vi "Path to L5K to import.vi"(8 "error in (no error)":errorcluster) -> (2 "Cancelled?":bool, 3 "Path to L5K file to import out":path)   [LabVIEW 2010, in "Ethernet IP Custom Device Custom Device.lvlib"]
doc: "Use this template to create a dialog box with event handling."
uses:
  Ethernet IP Custom Device Custom Device.lvlib
  <vilib>/NI VeriStand/Custom Device API/Custom Device Item Ref.ctl
  Ethernet IP Global Strings.vi
  <vilib>/NI Veristand/Custom Device API/Custom Device API.lvlib
panel:
  out "error out":errorcluster
  in  "Node Ptr":T1 format="%.0x"
  in  "Path to L5K file to import":path
  in  "Cancel":bool
  in  "OK":bool
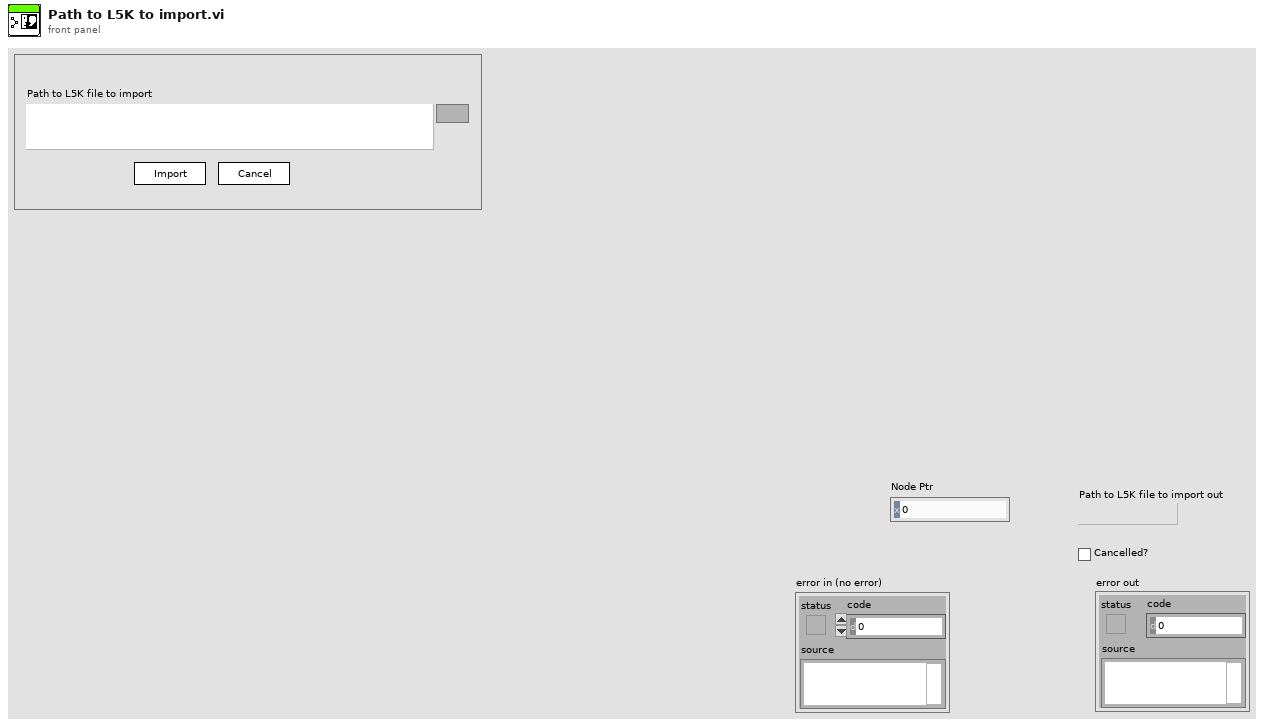
[diagram p1: front panel]
types:
  T1 = typedef "Custom Device API.lvlib/Custom Device Item Ref.ctl" = u64
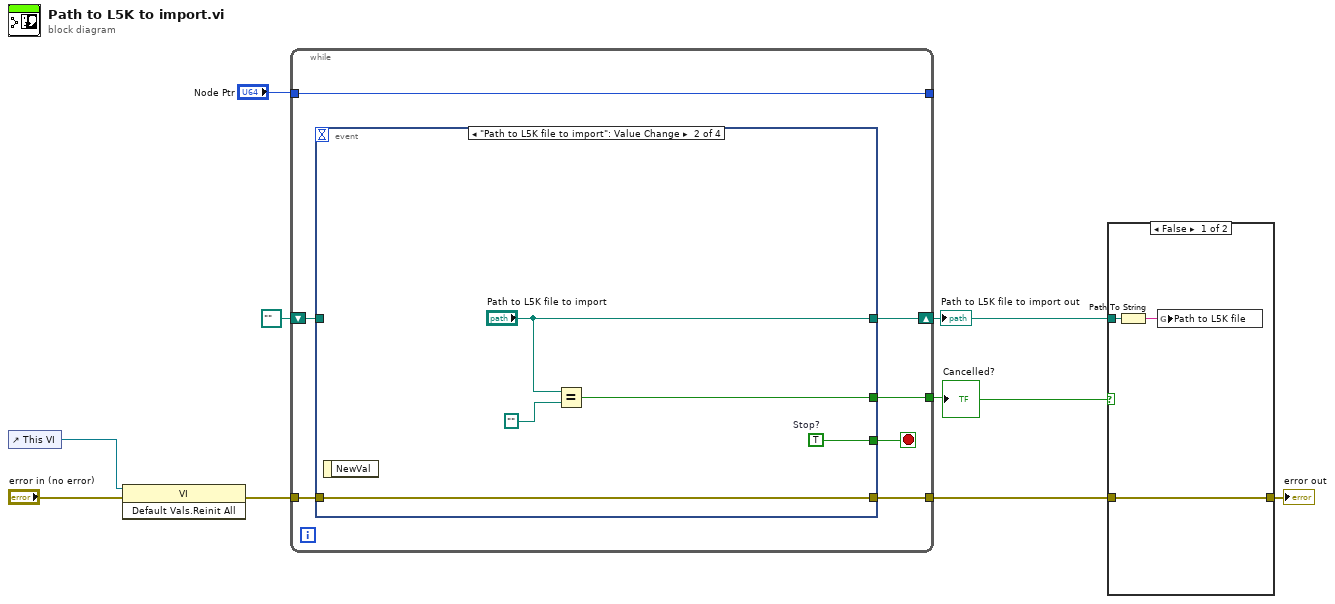
[diagram p0: block diagram]
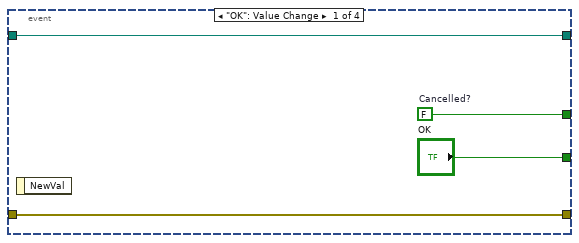
[diagram p3: hidden frame]
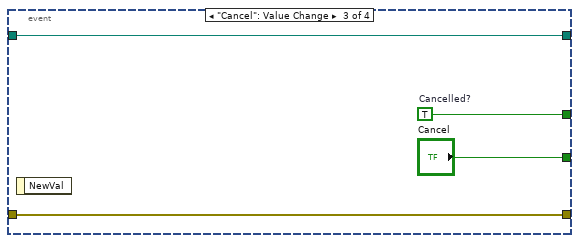
[diagram p4: hidden frame]
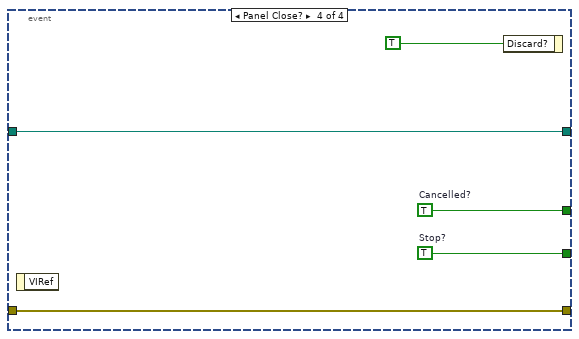
[diagram p5: hidden frame]
diagram:
  n1 = control-ref of="This VI"() -> (w8:refnum<vi>)
  n2 = invoke class="VI" method="Default Vals.Reinit All"(reference=w8, error in="error in (no error)") -> (error out=w7:errorcluster)  [unwired: 1 in, 2 out]
  n3 = while {
    tunnel: [w15] -> w4
    tunnel: w7 -> [w14]
    tunnel: [w13] -> w3
    shift-right: [w12] -> w1
    shift-left: path "" ("Path to L5K file to import") -> [w11]
    tunnel: "Node Ptr" -> [w10]
    tunnel: [w10] -> _
    stop <- w16 stop-if-true
    n4 = event shown="[1] \"Path to L5K file to import\": Value Change" {
      selector: _ -> [_ _ _ _]
      dyn-events: _ -> [_ _ _ _]
      timeout: _ -> [_ _ _ _]
      tunnel: ["OK" w23 "Cancel" w33] -> w16
      tunnel: [w20 w24 w29 w32] -> w15
      tunnel: w14 -> [w18 w22 w27 w31]
      tunnel: [w18 w22 w27 w31] -> w13
      tunnel: [w17 "Path to L5K file to import" w26 w30] -> w12
      tunnel: w11 -> [w17 _ w26 w30]
      event "OK": Value Change {
        w20 = FALSE  # Cancelled?
        n5 = event-data() -> ()  [unwired: 1 in, 1 out]
      }
      event "Path to L5K file to import": Value Change {
        w23 = TRUE  # Stop?
        n6 = event-data() -> ()  [unwired: 1 in, 1 out]
        n7 = Equal?(x="Path to L5K file to import", y=path "") -> (x = y?=w24:bool)
      }
      event "Cancel": Value Change {
        w29 = TRUE  # Cancelled?
        n8 = event-data() -> ()  [unwired: 1 in, 1 out]
      }
      event Panel Close? {
        w32 = TRUE  # Cancelled?
        w33 = TRUE  # Stop?
        n9 = event-data() -> ()  [unwired: 1 in, 1 out]
        n10 = event-data("Discard?"=TRUE) -> ()  [unwired: 1 in, 1 out]
      }
    }
  }
  "Cancelled?" <- w4
  "Path to L5K file to import out" <- w1
  n11 = case shown="False" w4 {
    tunnel: w3 -> [w36 w38]
    tunnel: [w36 w38] -> w2
    tunnel: w1 -> [w37 _]
    frame False {
      n12 = Path To String(path=w37) -> (string=w35:string)
      n13 = global write "Ethernet IP Global Strings.vi" "Path to L5K file"(w35) -> ()
    }
    frame True {
    }
  }
  "error out" <- w2
